vi "SetupDefault.vi"(8 "error in (no error)":errorcluster, 10 "Alias":string, 11 "SigGen_ESG in":refnum<class "SigGen_ESG.lvclass">) -> (0 "error out":errorcluster, 3 "SigGen_ESG out":refnum<class "SigGen_ESG.lvclass">)   [LabVIEW 2014, in "SigGen_ESG.lvclass"]
uses:
  SigGen_ESG.lvclass
  SigGen_ESG.lvclass/SigGen_ESG.ctl
  <instrlib>/Agilent ESG Series/Agilent ESG Series.lvlib
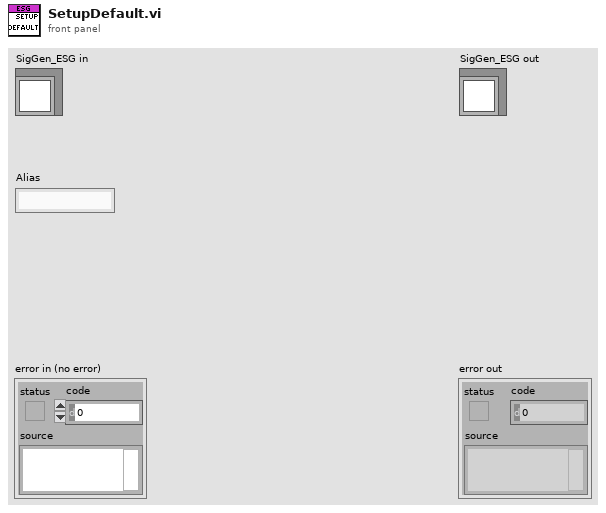
[diagram p1: front panel]
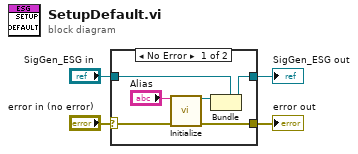
[diagram p0: block diagram]
diagram:
  n1 = case shown="No Error" "error in (no error)" {
    selector: "error in (no error)" -> [w10 w12]
    tunnel: "SigGen_ESG in" -> [w8 w11]
    tunnel: [w6 w11] -> w2
    tunnel: [w5 w12] -> w1
    frame No Error {
      n2 = call <instrlib>:"Initialize.vi"("VISA Resource Name"="Alias", "error in (no error)"=w10) -> ("VISA Resource Name Out"=w7:refnum<visa-resource-name>, "error out"=w5:errorcluster)  [unwired: 12 in]
      n3 = Bundle(cluster=w8, w7) -> (w6:refnum<class "SigGen_ESG.lvclass">)  [unwired: 1 in]
    }
    frame Error {
    }
  }
  "error out" <- w1
  "SigGen_ESG out" <- w2
